vi "SENS_SEGM_SWE_TIME_CONT_ON_OFF.vi"(0 "VISA IN":refnum<visa-resource-name>, 1 "Sweep Time Control ON/OFF":bool, 5 "error in":errorcluster, 7 "Channel":i32) -> (14 "VISA Out":refnum<visa-resource-name>, 19 "error out":errorcluster)   [LabVIEW 2018, in "PNA-X.lvlib"]
doc: "SENSe<cnum>:SEGMent:SWEep:TIME:CONTrol <ON | OFF> \n1813\n\n(Read-Write) Specifies whether Sweep Time can be set independently for each sweep segment. \nParameters \n<cnum> Any existing channel number. If unspecified, value is set to 1 \n<ON | OFF> ON (or 1) - turns Sweep Time control ON. Sweep Time can be set for each \nsegment. \nOFF (or 0) - turns Sweep Time control OFF. Uses the channel Sweep Time \nsetting. \nExamples SENS:SEGM:SWE:TIM:CONT ON \nsense2:segment:sweep:time:control off \nQuery Syntax SENSe<cnum>:SEGMent:SWEep:TIME:CONTrol? \nReturn Type Boolean (1 = ON, 0 = OFF) \nDefault OFF"
uses:
  PNA-X.lvlib
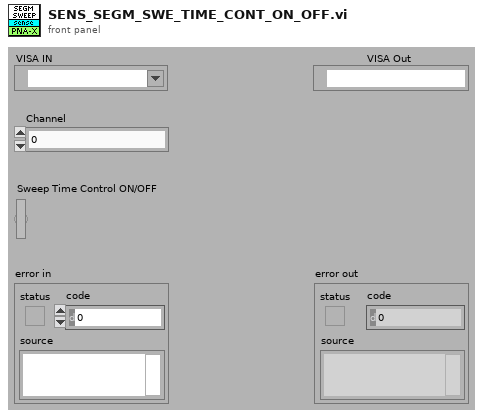
[diagram p1: front panel]
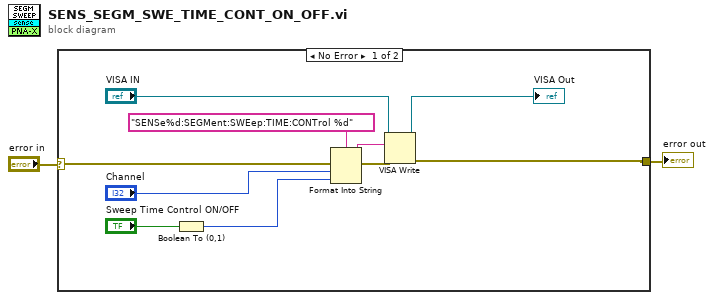
[diagram p0: block diagram]
diagram:
  n1 = case shown="No Error" "error in" {
    selector: "error in" -> [w12 w13]
    tunnel: [w7 w13] -> w1
    frame No Error {
      n2 = Boolean To (0,1)(Boolean="Sweep Time Control ON/OFF") -> (0, 1=w3:i16)
      n3 = Format Into String(format string="SENSe%d:SEGMent:SWEep:TIME:CONTrol %d" ("Cmdline"), error in=w12, "Channel", w3) -> (resulting string=w10:string, error out=w11:errorcluster)  [unwired: 1 in]
      n4 = VISA Write(VISA resource name="VISA IN", write buffer=w10, error in (no error)=w11) -> (VISA resource name out=→"VISA Out":refnum<visa-resource-name>, error out=w7:errorcluster)  [unwired: 1 out]
    }
    frame Error {
    }
  }
  "error out" <- w1
